vi "SDL Shutdown.vi"(8 "error in (no error)":errorcluster, 11 "Main Controller Actor in":refnum<class "Main Controller Actor.lvclass">) -> (0 "error out":errorcluster, 3 "Main Controller Actor out":refnum<class "Main Controller Actor.lvclass">)   [LabVIEW 2021, in "Main Controller Actor.lvclass"]
uses:
  Main Controller Actor.lvclass
  Main Controller Actor.lvclass/Main Controller Actor.ctl
  LabSDL2/Source/Libraries/LibSDL2 Wrapper/LibSDL2.lvlib
  LabSDL2/Source/Libraries/LibSDL2_Image Wrapper/LibSDL2_Image.lvlib
  LabSDL2/Source/Libraries/LibSDL2_Mixer Wrapper/LibSDL2_Mixer.lvlib
  LabSDL2/Source/Libraries/LibSDL2_TTF Wrapper/LibSDL2_TTF.lvlib
  Renderer/Renderer.lvclass
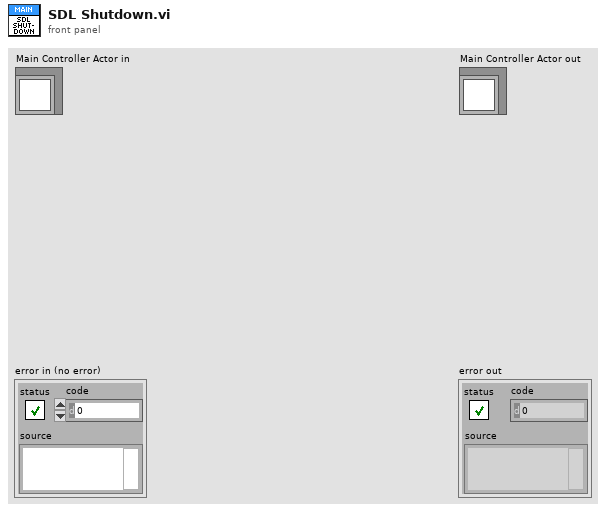
[diagram p1: front panel]
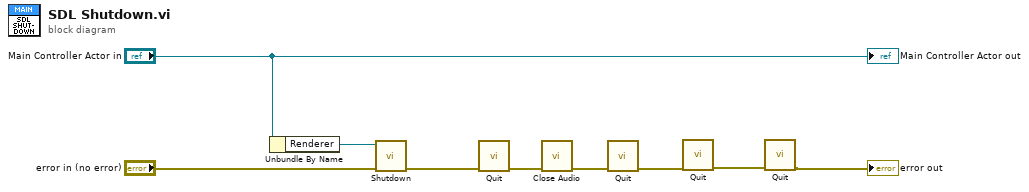
[diagram p0: block diagram]
diagram:
  n1 = Unbundle By Name("Main Controller Actor in") -> ("Renderer"=w1:refnum<class "Renderer.lvclass">)
  n2 = call "Shutdown.vi"("error in (no error)"="error in (no error)", "Renderer"=w1) -> ("error out"=w2:errorcluster)  [unwired: 9 in]
  n3 = call "Quit.vi"("error in (no error)"=w2) -> ("error out"=w9:errorcluster)  [unwired: 10 in]
  n4 = call "Close Audio.vi"("error in"=w9) -> ("error out"=w7:errorcluster)  [unwired: 10 in]
  n5 = call "Quit.vi"("error in"=w7) -> ("error out"=w8:errorcluster)  [unwired: 10 in]
  n6 = call "Quit.vi"("error in"=w8) -> ("error out"=w6:errorcluster)  [unwired: 10 in]
  n7 = call "Quit.vi"("error in"=w6) -> ("error out"=→"error out":errorcluster)  [unwired: 10 in]
  "Main Controller Actor out" <- "Main Controller Actor in"
